vi "GT Get Laser Follow Spline.vi"(0 "cardNum":i16, 1 "tableId":i16, 2 "n":i32, 3 "pX":dbl, 4 "pY":dbl, 5 "pA":dbl, 6 "pB":dbl, 7 "error in (no error)":errorcluster caption="错误输入（无错误）", 8 "pC":dbl, 9 "pCount":i32, 10 "channel":i16) -> (18 "pC out":dbl, 19 "pCount out":i32, 20 "function return":i16, 23 "pX out":dbl, 24 "pY out":dbl, 25 "pA out":dbl, 26 "pB out":dbl, 27 "error out":errorcluster caption="错误输出")   [LabVIEW 2014, in "gts.lvlib"]
doc: "GT_API GT_GetLaserFollowSpline(short cardNum,short tableId,long n,double *pX,double *pY,double *pA,double *pB,double *pC,long *pCount,short channel=0);"
uses:
  gts.lvlib
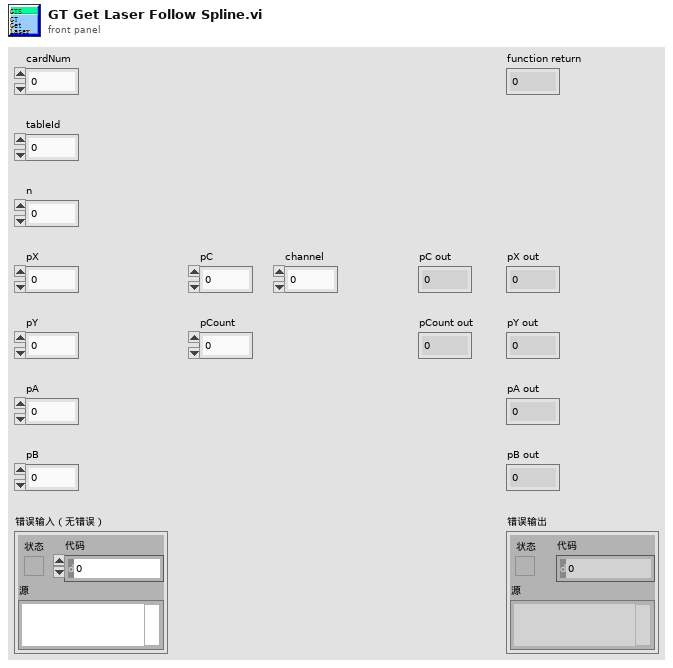
[diagram p1: front panel]
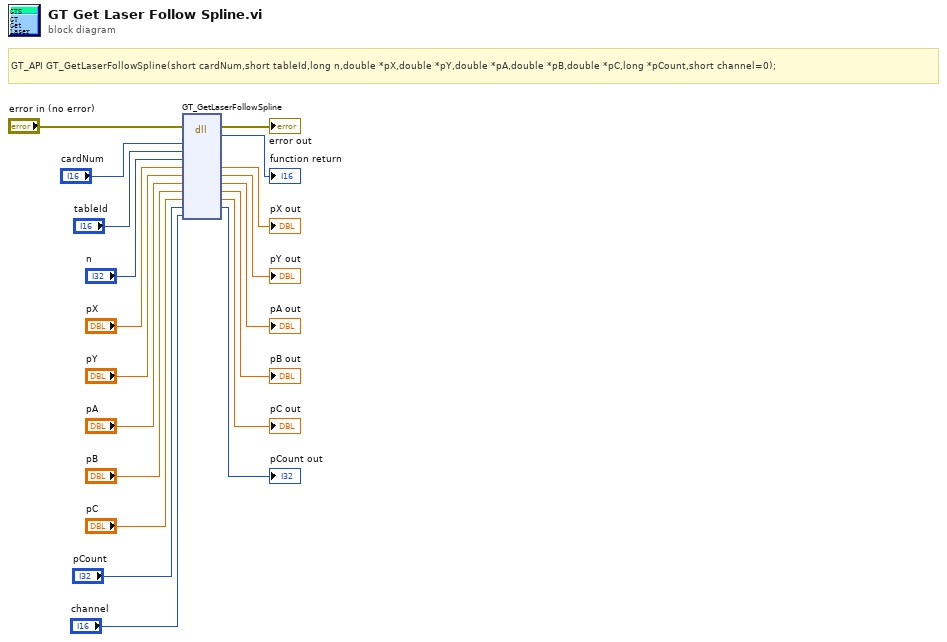
[diagram p0: block diagram]
diagram:
  # "GT_API GT_GetLaserFollowSpline(short cardNum,short tableId,long n,double *pX,double *pY,double *pA,double *pB,double *pC,long *pCount,short channel=0);"
  n1 = dll-call lib="PTH2habs D固高科技资料GTS控制卡GTS卡18年上半年资料dllVC32bit\nmulti_cardgts.*" fn="GT_GetLaserFollowSpline"(error in="error in (no error)", "cardNum"="cardNum", "tableId"="tableId", "n"="n", "pX"="pX", "pY"="pY", "pA"="pA", "pB"="pB", "pC"="pC", "pCount"="pCount", "channel"="channel") -> (error out=→"error out":errorcluster, →"function return":i16, "pX"=→"pX out":dbl, "pY"=→"pY out":dbl, "pA"=→"pA out":dbl, "pB"=→"pB out":dbl, "pC"=→"pC out":dbl, "pCount"=→"pCount out":i32)  [unwired: 6 in, 1 out]
